vi "OpenCOMPort.vi"(8 "error in (no error)":errorcluster, 10 "COM port parameters":T1={"Port ID"=2, "Baud rate"=38400, "Data bits"=8, "Parity"=enum."None", "Stop bits"=1.0, "Flow control"=enum."None"} {"Stop bits" items=["1"=1.0, "1.5"=1.5, "2"=2.0]; "Data bits" items=["5"=5, "6"=6, "7"=7, "8"=8]; "Baud rate" items=["110"=110, "300"=300, "1200"=1200, "2400"=2400, "4800"=4800, "9600"=9600, "19200"=19200, "38400"=38400, "57600"=57600, "115200"=115200, "128000"=128000, "256000"=256000]; "Port ID" items=["COM2"=2, "COM3"=3]}, 11 "SM1000-control in":T2) -> (0 "error out":errorcluster, 3 "SM1000-control out":T2)   [LabVIEW 2013, in "HardwareCharacterization.lvlib" / "HC-SM1000.lvclass"]
doc: "Opens the specified serial I/O COM port on the EC1000.\n\nThis command is available only if the system is configured for accepting streaming job data over Ethernet.\nThe specified COM port is opened and is available for serial I/O.\nThis operation is intended to permit out-of-band communication to serial port based automation devices or laser systems.\nA normal configuration might be specified as: \"OpenCOMPort,2,38400,8,None,1,None.\nOnly COM port-ID 1 has hardware flow control support.\n\nCommand: <\"OpenCOMPort\">,<port-ID>,<baud-rate>,<data-bits>,<parity>,<stop-bits>,<flow-control> or 14,<port-ID>,<baud-rate>,<data-bits>,<parity>,<stop-bits>,<flow-control>\nReturns: \"0\""
uses:
  HC-SM1000.lvclass
  Object-reference.ctl
  COM-parameters.ctl
  HC-SM1000.lvclass/HC-SM1000.ctl
  Custom-errors.ctl
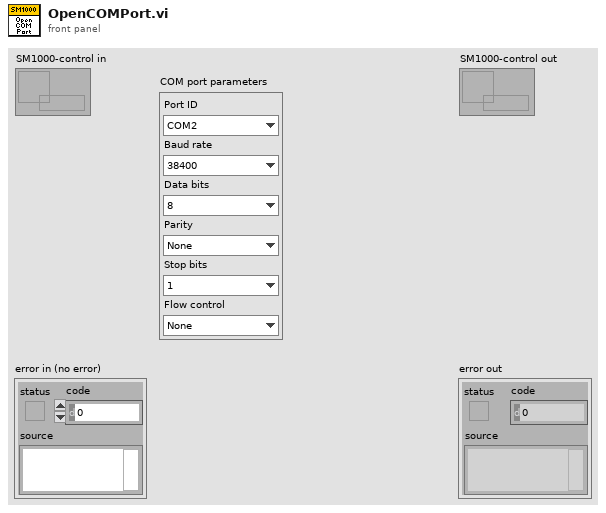
[diagram p1: front panel]
types:
  T1 = typedef "HardwareCharacterization.lvlib/HC-SM1000.lvclass/COM-parameters.ctl" = cluster{"Port ID":i32, "Baud rate":i32, "Data bits":i32, "Parity":enum16{"Even", "Odd", "None", "Mark", "Space"}, "Stop bits":dbl, "Flow control":enum16{"None", "XonXoff", "CTS_RTS", "DSR_DTR"}}
  T2 = typedef "HardwareCharacterization.lvlib/HC-SM1000.lvclass/Object-reference.ctl" = refnum<data-value>
  T3 = typedef "HardwareCharacterization.lvlib/HC-SM1000.lvclass/Custom-errors.ctl" = enum16{"No error", "Not implemented", "Command not recognized", "Invalid input", "No connection", "Timeout", "Resource not loaded"}
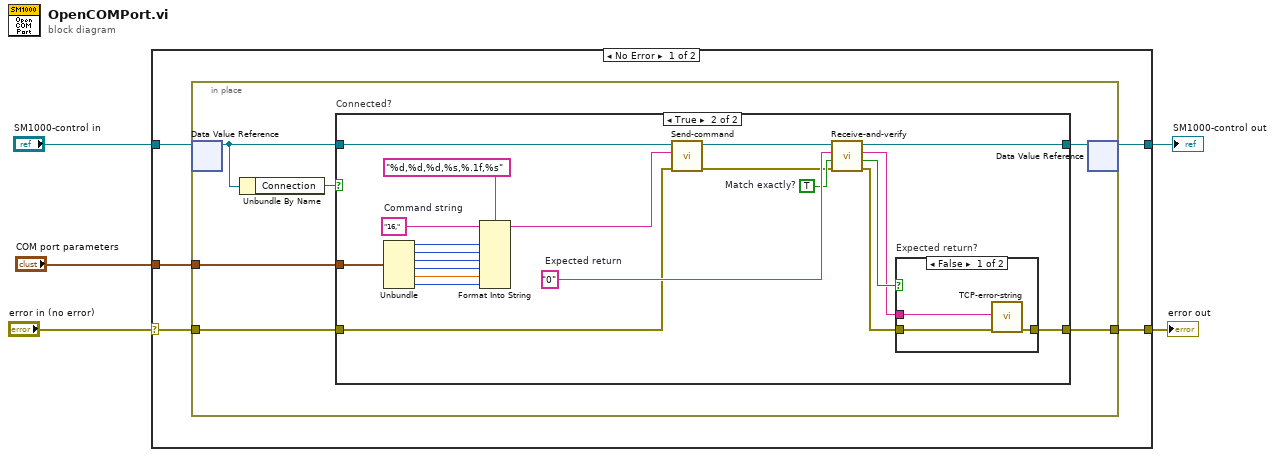
[diagram p0: block diagram]
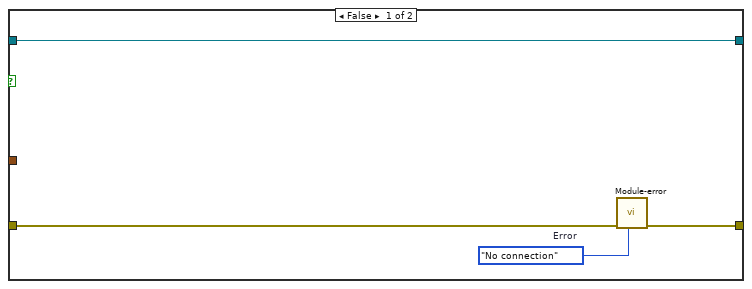
[diagram p2: hidden frame]
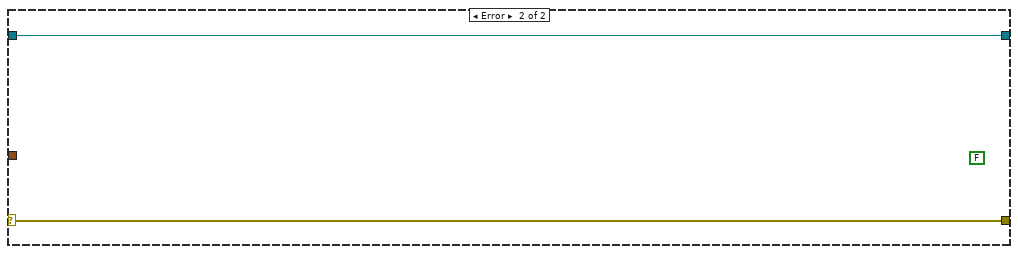
[diagram p4: hidden frame]
diagram:
  n1 = case shown="No Error" "error in (no error)" {
    selector: "error in (no error)" -> [w8 w47]
    tunnel: [w7 w47] -> w4
    tunnel: [w9 w46] -> w2
    tunnel: "SM1000-control in" -> [w10 w46]
    tunnel: "COM port parameters" -> [w6 _]
    frame No Error {
      n2 = in-place {
        in-place-border: w8 -> [w16]
        in-place-border: [w13] -> w7
        in-place-border: w6 -> [w11]
        n3 = in-place-dvr #1(w10) -> (w14:refnum<class "HC-SM1000.lvclass">)  [unwired: 1 out]
        n4 = Unbundle By Name(w14) -> ("Connection"=w15:bool)
        n5 = case "Connected?" shown="True" w15 {
          tunnel: w16 -> [w20 w34]
          tunnel: w14 -> [w18 w41]
          tunnel: [w19 w32] -> w13
          tunnel: [w18 w31] -> w12
          tunnel: w11 -> [_ w29]
          frame False {
            w17 = Custom-errors."No connection"  # Error
            n6 = call "Module-error.vi"("Error"=w17, "error in (no error)"=w20) -> ("error out"=w19:errorcluster)  [unwired: 9 in]
          }
          frame True {
            w38 = TRUE  # Match exactly?
            w39 = "0"  # Expected return
            w30 = "16,"  # Command string
            n7 = Unbundle(w29) -> ("Port ID"=w28:i32, "Baud rate"=w27:i32, "Data bits"=w26:i32, "Parity"=w25:enum16{"Even", "Odd", "None", "Mark", "Space"}, "Stop bits"=w24:dbl, "Flow control"=w23:enum16{"None", "XonXoff", "CTS_RTS", "DSR_DTR"})
            n8 = Format Into String(format string="%d,%d,%d,%s,%.1f,%s", initial string=w30, w28, w27, w26, w25, w24, w23) -> (resulting string=w21:string)  [unwired: 1 in, 1 out]
            n9 = call "Send-command.vi"("error in (no error)"=w34, "Command string"=w21, "SM1000-control in"=w41) -> ("error out"=w37:errorcluster, "SM1000-control out"=w40:refnum<class "HC-SM1000.lvclass">)  [unwired: 7 in]
            n10 = call "Receive-and-verify.vi"("error in (no error)"=w37, "Match exactly?"=w38, "Expected return string"=w39, "SM1000-control in"=w40) -> ("error out"=w33:errorcluster, "Verified?"=w36:bool, "Return string"=w35:string, "SM1000-control out"=w31:refnum<class "HC-SM1000.lvclass">)  [unwired: 4 in]
            n11 = case "Expected return?" shown="False" w36 {
              tunnel: w35 -> [w44 _]
              tunnel: w33 -> [w43 w45]
              tunnel: [w42 w45] -> w32
              frame False {
                n12 = call "TCP-error-string.vi"("error in (no error)"=w43, "Retun code"=w44) -> ("error out"=w42:errorcluster)  [unwired: 9 in]
              }
              frame True {
              }
            }
          }
        }
        n13 = in-place-dvr #1(w12) -> (w9:T2)  [unwired: 1 out]
      }
    }
    frame Error {
      (unwired) FALSE
    }
  }
  "error out" <- w4
  "SM1000-control out" <- w2
